vi "1D_tipconvolution.vi"() -> ()   [LabVIEW 2017]
panel:
  in  "stop":bool
  in  "angle":dbl=35.0 min=1.0 max=89.0 format="%.2f"
  in  "radius of curvature":dbl=50.0 min=1.0 max=1000.0 format="%.2f"
  in  "height":dbl=120.0 format="%.2f"
  in  "Show tip?":bool=TRUE
  in  "Show sample":bool=TRUE
  in  "scanning speed":u32(slide)=66 scale=1.0..1000.0
  in  "slope":dbl=1.0 format="%.2f"
  out "Waveform Graph":dbl[][](graph)
  in  "width":dbl=140.0 format="%.2f"
  in  "period":dbl=310.0 format="%.2f"
  # "tipdefinition"
  # "sampleshape"
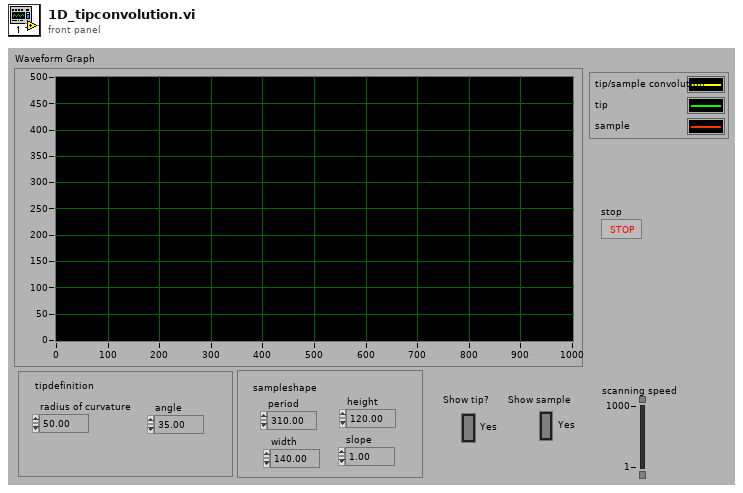
[diagram p1: front panel]
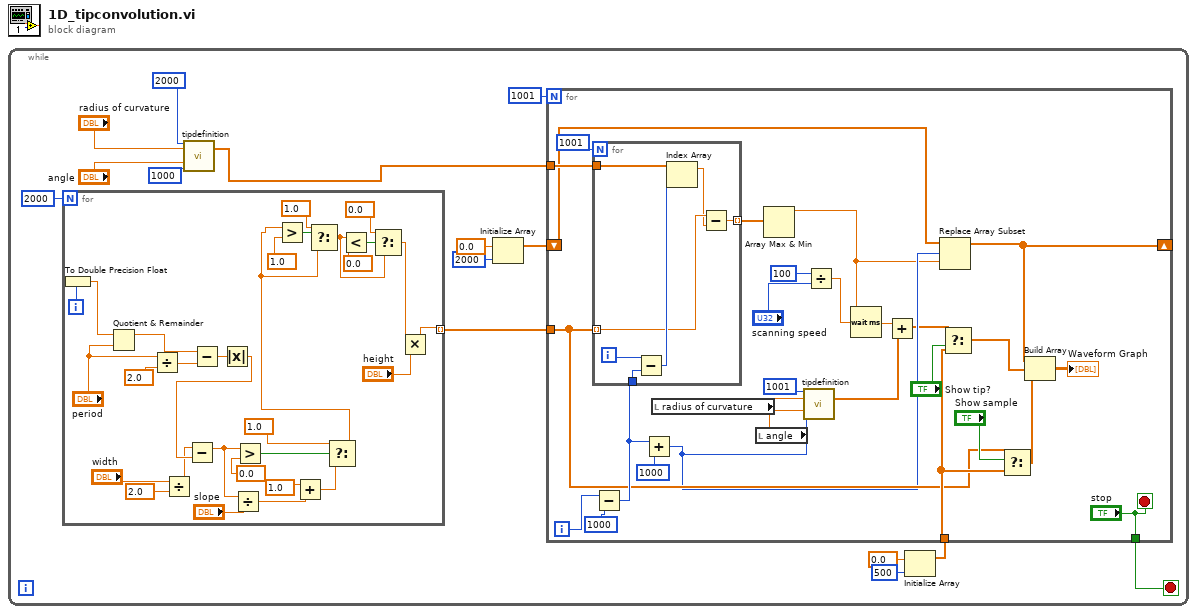
[diagram p0: block diagram]
diagram:
  n1 = while {
    stop <- w1 stop-if-true
    n2 = for {
      N: 2000 -> [_]
      tunnel: [w51] -> w13 mode=indexing
      i -> [w79]
      n3 = To Double Precision Float(number=w79) -> (double precision float=w50:dbl)
      n4 = Quotient & Remainder(x=w50, y="period") -> (x-y*floor(x/y)=w68:dbl)  [unwired: 1 out]
      n5 = Divide(x="period", y=2.0) -> (x/y=w67:dbl)
      n6 = Divide(x="width", y=2.0) -> (x/y=w63:dbl)
      n7 = Subtract(x=w68, y=w67) -> (x-y=w66:dbl)
      n8 = Absolute Value(x=w66) -> (abs(x)=w64:dbl)
      n9 = Subtract(x=w63, y=w64) -> (x-y=w57:dbl)
      n10 = Divide(x=w57, y="slope") -> (x/y=w56:dbl)
      n11 = Greater?(x=w57, y=0.0) -> (0:w61:bool)
      n12 = Add(x=1.0, y=w56) -> (x+y=w55:dbl)
      n13 = Select(t=1.0, s=w61, f=w55) -> (s? t:f=w54:dbl)
      n14 = Greater?(x=w54, y=1.0) -> (0:w74:bool)
      n15 = Select(t=1.0, s=w74, f=w54) -> (s? t:f=w69:dbl)
      n16 = Less?(x=w69, y=0.0) -> (x < y?=w71:bool)
      n17 = Select(t=0.0, s=w71, f=w69) -> (s? t:f=w52:dbl)
      n18 = Multiply(x=w52, y="height") -> (x*y=w51:dbl)
    }
    n19 = call "tipdefinition.vi"("#points"=2000, "radius of curvature"="radius of curvature", "tipangle"="angle", "offset"=1000) -> ("output"=w4:dbl[])  [unwired: 11 in]
    n20 = Initialize Array(0.0 ("Element Data"), 2000 ("Dimension Size")) -> (w12:dbl[])
    n21 = Initialize Array(0.0 ("Element Data"), 500 ("Dimension Size")) -> (w7:dbl[])
    n22 = for {
      N: 1001 -> [_]
      tunnel: w13 -> [w29]
      tunnel: w4 -> [w41]
      shift-right: [w34] -> _
      shift-left: w12 -> [w37]
      tunnel: w7 -> [w30]
      tunnel: ["stop"] -> w1
      i -> [w39]
      stop <- "stop" stop-if-true
      n23 = Subtract(x=w39, y=1000) -> (x-y=w35:i32)
      n24 = for {
        N: 1001 -> [_]
        tunnel: w29 -> [w45] mode=indexing
        tunnel: w35 -> [w43]
        tunnel: w41 -> [w48]
        tunnel: [w46] -> w40 mode=indexing
        i -> [w49]
        n25 = Subtract(x=w49, y=w43) -> (x-y=w47:i32)
        n26 = Index Array(array=w48, index=w47) -> (element=w44:dbl)
        n27 = Subtract(x=w45, y=w44) -> (x-y=w46:dbl)
      }
      n28 = Add(x=w35, y=1000) -> (x+y=w23:i32)
      n29 = local read "radius of curvature"() -> (w20:dbl)
      n30 = local read "angle"() -> (w19:dbl)
      n31 = Array Max & Min(array=w40) -> (max value=w22:dbl)  [unwired: 3 out]
      n32 = call "tipdefinition.vi"("#points"=1001, "radius of curvature"=w20, "tipangle"=w19, "offset"=w23) -> ("output"=w18:dbl[])  [unwired: 11 in]
      n33 = Divide(x=u32 100, y="scanning speed") -> (x/y=w26:dbl)
      n34 = Wait (ms)(milliseconds to wait=w26) -> ()  [unwired: 1 out]
      n35 = Add(x=w22, y=w18) -> (x+y=w17:dbl[])
      n36 = Replace Array Subset(array=w37, new element=w22, index=w23) -> (w34:dbl[])
      n37 = Select(t=w17, s="Show tip?", f=w30) -> (s? t:f=w32:dbl[])
      n38 = Select(t=w29, s="Show sample", f=w30) -> (s? t:f=w28:dbl[])
      n39 = Build Array(w34, w32, w28) -> (→"Waveform Graph":dbl[][])
    }
  }
